vi "In_S6F19.vi"(8 "error in (no error)":errorcluster, 11 "S6 Message Class in":refnum<class "S6 Message Class.lvclass">) -> (0 "error out":errorcluster, 1 "OK?":bool, 2 "RPTID":u32, 3 "S6 Message Class out":refnum<class "S6 Message Class.lvclass">)   [LabVIEW 2020, in "SECS Communication.lvlib" / "S6 Message Class.lvclass"]
uses:
  S6 Message Class.lvclass
  D:/Dropbox/SECS/SECS_GEM v1.0.6/Com/SECS Communication/SECS-II Class/SECS-II Class.lvclass
  SECS-II Class/SECS-II Class.lvclass/SECS-II Class.ctl
  SECS-II Class/Variant To Data_U4.vi
  SECS-II Class/SECS-II Class.lvclass
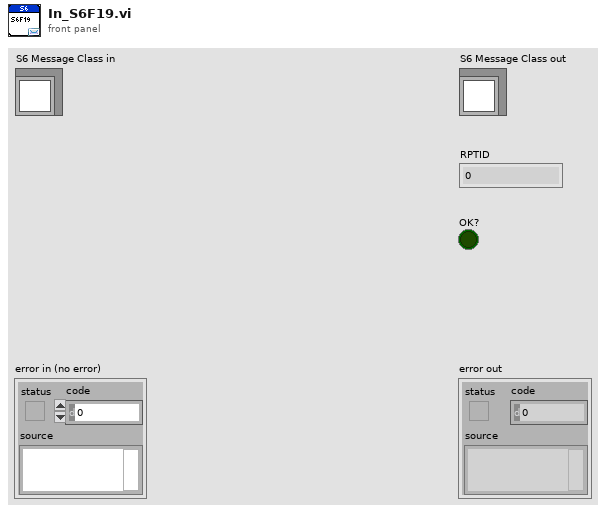
[diagram p1: front panel]
types:
  T1 = typedef "SECS Communication.lvlib/SECS-II Class.lvclass/Message Data.ctl" = cluster{"Index":i32, "Data Item Format":T2, "Format Code":T3, "Parent Index":i32, "Child Index":i32[], "Data":variant}
  T2 = typedef "SECS Communication.lvlib/SECS-II Class.lvclass/Data Item Format.ctl" = enum16{"Data Type", "Value"}
  T3 = typedef "SECS Communication.lvlib/SECS-II Class.lvclass/Format Code.ctl" = enum16{"L", "A", "B", "Boolean", "J", "I1", "I2", "I4", "I8", "U1", "U2", "U4", "U8", "F4", "F8", "Char"}
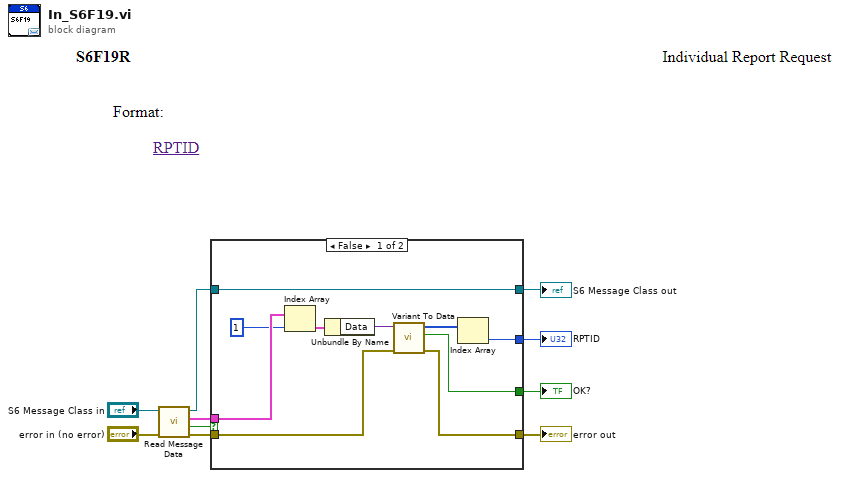
[diagram p0: block diagram]
diagram:
  n1 = call "Read Message Data.vi"("error in (no error)"="error in (no error)", "SECS-II Class in"="S6 Message Class in") -> ("error out"=w9:errorcluster, "Empty?"=w4:bool, "Message Data"=w10:T1[], "SECS-II Class out"=w3:refnum<class "S6 Message Class.lvclass">)  [unwired: 6 in]
  n2 = case shown="False" w4 {
    tunnel: w10 -> [w20 _]
    tunnel: w9 -> [w16 w22]
    tunnel: [w14 _] -> w6
    tunnel: [w13 w22] -> w5
    tunnel: w3 -> [w12 w21]
    tunnel: [w12 w21] -> w2
    tunnel: [w11 _] -> w1
    frame False {
      n3 = Index Array(array=w20, index=1) -> (element=w18:T1)
      n4 = Unbundle By Name(w18) -> ("Data"=w17:variant)
      n5 = call-poly "Variant To Data.vi"("error in (no error)"=w16, "Variant"=w17) -> ("error out"=w13:errorcluster, "OK?"=w11:bool, "Data"=w15:u32[])  [unwired: 7 in]
      n6 = Index Array(array=w15) -> (element=w14:u32)  [unwired: 1 in]
    }
    frame True {
    }
  }
  "error out" <- w5
  "S6 Message Class out" <- w2
  "RPTID" <- w6
  "OK?" <- w1
